vi "IsColumn1Section3Header.vi"(8 "error in (no error)":errorcluster, 9 "index 3":i32, 10 "index 2":i32, 11 "index 1":i32) -> (0 "error out":errorcluster, 3 "is col 1 section 3 header?":bool)   [LabVIEW 2009, in "NavScreen.lvlib"]
uses:
  NavScreen.lvlib
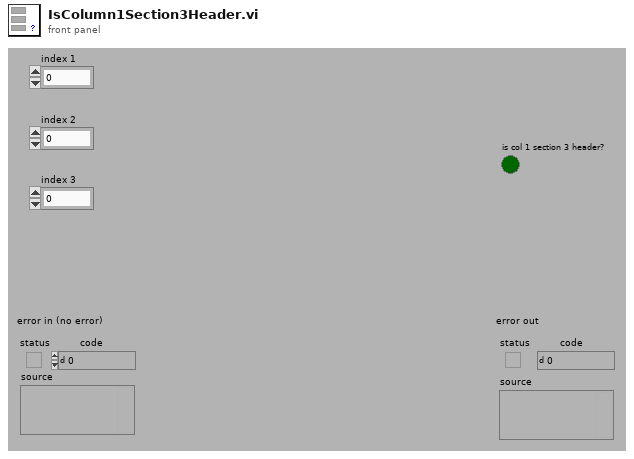
[diagram p1: front panel]
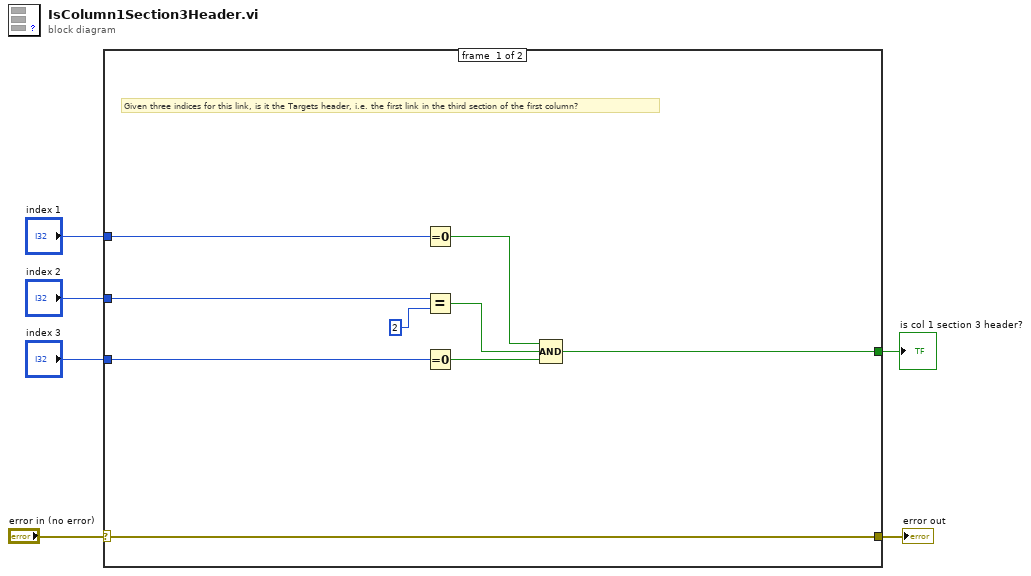
[diagram p0: block diagram]
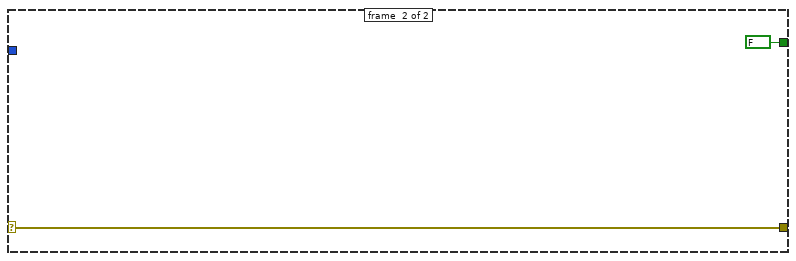
[diagram p2: hidden frame]
diagram:
  n1 = case shown="No Error" "error in (no error)" {
    selector: "error in (no error)" -> [w15 w17]
    tunnel: [w15 w17] -> w5
    tunnel: "index 1" -> [w14 _]
    tunnel: "index 2" -> [w12 _]
    tunnel: "index 3" -> [w9 _]
    tunnel: [w7 FALSE] -> w1
    frame #0 {
      # "Given three indices for this link, is it the Targets header, i.e. the first link in the third section of the first column?"
      n2 = Equal To 0?(x=w14) -> (x = 0?=w13:bool)
      n3 = Equal?(x=w12, y=2) -> (x = y?=w10:bool)
      n4 = Equal To 0?(x=w9) -> (x = 0?=w8:bool)
      n5 = Compound Arithmetic op=AND(w13, w10, w8) -> (w7:bool)
    }
    frame #1 {
    }
  }
  "error out" <- w5
  "is col 1 section 3 header?" <- w1
